vi "WPI_CANTalonSRX_Receive.vi"(11 "Device ID (0)":u8) -> (3 "Device ID":u8)   [LabVIEW 2016]
uses:
  <vilib>/Rock Robotics/WPI/ThirdParty/CanMotor/TalonSRX/WPI_CANTalonSRX_MessageIDs.ctl
  <vilib>/Rock Robotics/WPI/ThirdParty/CanMotor/TalonSRX/WPI_CANTalonSRX_GlobalOps.ctl
  <vilib>/Rock Robotics/WPI/ThirdParty/CanMotor/TalonSRX/WPI_CANTalonSRX_GlobalStatus.ctl
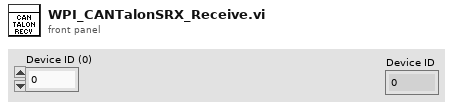
[diagram p1: front panel]
types:
  T1 = typedef "WPI_CANTalonSRX_MessageIDs.ctl" = u32
  T2 = typedef "WPI_CANTalonSRX_GlobalStatus.ctl" = cluster{"Applied Throttle":dbl, "Module Enabled":bool, "CAN Error":errorcluster, "Closed Loop Error":dbl, "Forward Limit Switch Closed":bool, "Reverse Limit Switch Closed":bool, "Sensor Position":dbl, "Sensor Velocity":dbl, "Current":dbl, "Sticky Fault - Over Temp":bool, "Sticky Fault - Under Voltage":bool, "Sticky Fault - Forward Limit":bool, "Sticky Fault - Reverse Limit":bool, "Sticky Fault - Forward Soft Limit":bool, "Sticky Fault - Reverse Soft Limit":bool, "Brake is Enabled":bool, "Encoder Position":dbl, "Encoder Velocity":dbl, "Encoder Index Count":dbl, "Encoder A Pin State":bool, "Encoder B Pin State":bool, "Encoder Index Pin State":bool, "Analog In":dbl, "Analog In Velocity":dbl, "Temperature (C)":dbl, "Battery Voltage":dbl, "Control 5 Is Supported":bool, "Current Profile Slot Select":dbl, "Pos Div 8":bool, "Vel Div 4":bool, "Pulse Width Position":i32, "Pulse Width Velocity":i32, "Pulse Width Rise To Rise (us)":i32, "Pulse Width Rise To Fall (us)":i32, "Mot Prof Active Is Under Run":bool, "Mot Prof Active Has Under Run":bool, "Mot Prof Active Is Last":bool, "Mot Prof Active Velocity Only":bool, "Mot Prof Active Is Valid":bool, "Mot Prof Buffer Is Full":bool, "Mot Prof Active Profile Slot Select":i32, "Mot Prof NextID":i32, "Mot Prof Count":i32, "Mot Prof Active Velocity":dbl, "Mot Prof Active Position":dbl, "Mot Prof Output Enable":i32, "UsageFrame":u32, "Motion Magic Active Trajectory":cluster{"Velocity":dbl, "Position":dbl}}
  T3 = typedef "WPI_CANTalonSRX_GlobalOps.ctl" = enum16{"Read For Send", "Write After Receive General", "Write After Receive Feedback", "Write After Receive Encoder", "Write After Receive Ain", "Write Error", "Get All", "Set Output", "Set Mode", "Set Master ID", "Set Brake Mode", "Set Reverse Feedback Sensor", "Set Reverse Closed Loop Output", "Set Override Limits", "Set Forward Limit Enabled", "Set Reverse Limit Enabled", "Set Feedback Select", "Set Profile Select", "Set Throttle Ramp Rate", "Disable", "Set Enc Codes Per Rev", "Set Num Pot Turns", "Set Control Frame Rate", "Enable Legacy Control", "Write After Receive Pulse Width", "Set Enable Frame Rate", "Write After Receive Motion Profile", "Set Motion Profile Flow Control", "Set Motion Profile Control Frame Rate", "Set Current Limit Enable", "Set Usage Frame", "Write After Receive Motion Magic"}
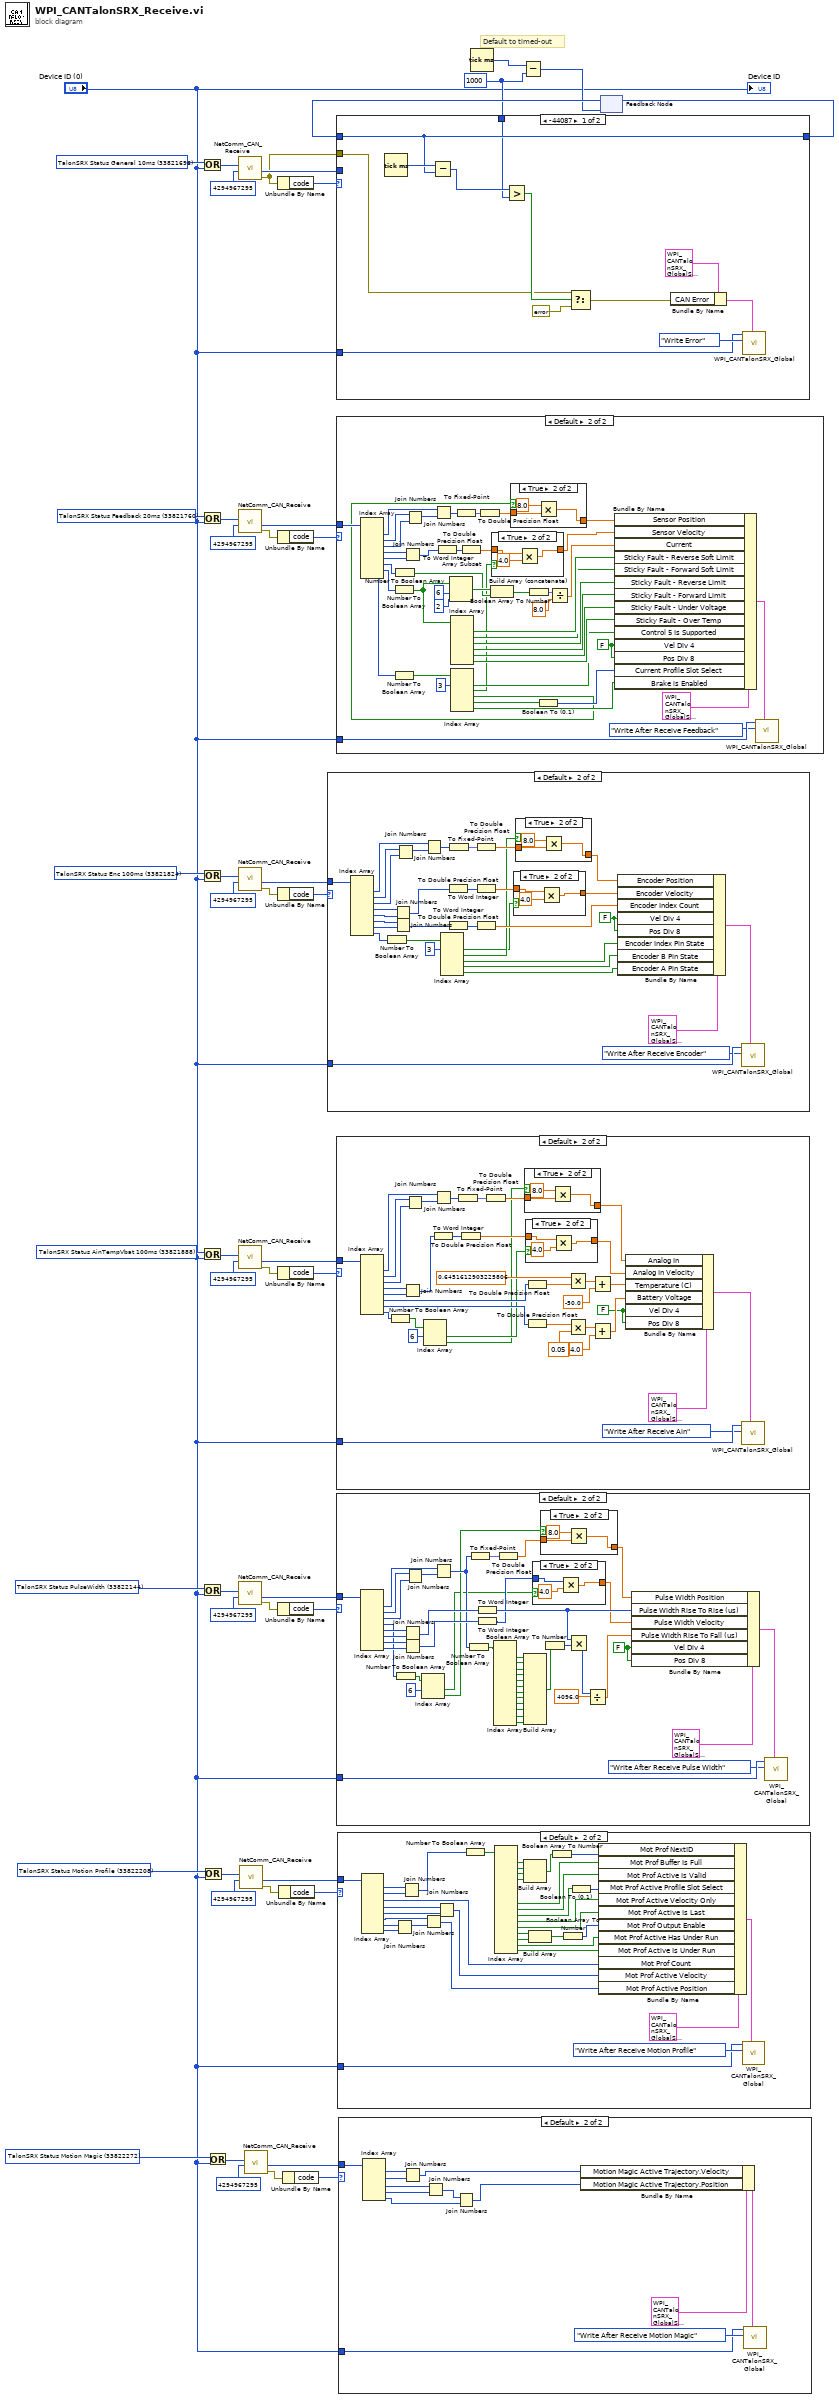
[diagram p0: block diagram]
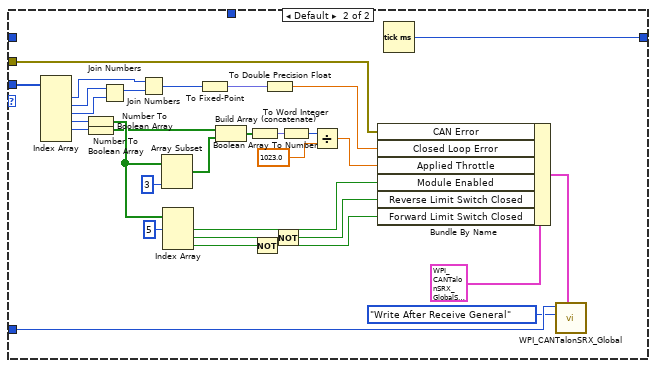
[diagram p16: hidden frame]
diagram:
  w2 = T1 33822272 items=["TalonSRX Control General 10ms"=33816576, "TalonSRX Control Rates Slow"=33816640, "TalonSRX Control ClearFlags Slow"=33816704, "TalonSRX Status General 10ms"=33821696, "TalonSRX Status Feedback 20ms"=33821760, "TalonSRX Status Enc 100ms"=33821824, "TalonSRX Status AinTempVbat 100ms"=33821888, "TalonSRX Status Startup Once"=33821952, "TalonSRX Status Debug"=33822080, "TalonSRX Config SetGainsSlot0 A"=33823808, "TalonSRX Config SetGainsSlot0 B"=33823872, "TalonSRX Config SetGainsSlot1 A"=33823936, "TalonSRX Config SetGainsSlot1 B"=33824000, "TalonSRX Config SetSoftLimits"=33824064, "TalonSRX Config WebControl"=33824128, "TalonSRX Param Request"=33822720, "TalonSRX Param Response"=33822784, "TalonSRX Param Set"=33822848, "TalonSRX Status PulseWidth"=33822144, "TalonSRX Status Motion Profile"=33822208, "TalonSRX Control General 5"=33816832, "TalonSRX Control Motion Profile Add"=33816896, "TalonSRX Status Motion Magic"=33822272] ("Talon SRX Control Frame")
  w8 = T1 33822208 items=["TalonSRX Control General 10ms"=33816576, "TalonSRX Control Rates Slow"=33816640, "TalonSRX Control ClearFlags Slow"=33816704, "TalonSRX Status General 10ms"=33821696, "TalonSRX Status Feedback 20ms"=33821760, "TalonSRX Status Enc 100ms"=33821824, "TalonSRX Status AinTempVbat 100ms"=33821888, "TalonSRX Status Startup Once"=33821952, "TalonSRX Status Debug"=33822080, "TalonSRX Config SetGainsSlot0 A"=33823808, "TalonSRX Config SetGainsSlot0 B"=33823872, "TalonSRX Config SetGainsSlot1 A"=33823936, "TalonSRX Config SetGainsSlot1 B"=33824000, "TalonSRX Config SetSoftLimits"=33824064, "TalonSRX Config WebControl"=33824128, "TalonSRX Param Request"=33822720, "TalonSRX Param Response"=33822784, "TalonSRX Param Set"=33822848, "TalonSRX Status PulseWidth"=33822144, "TalonSRX Status Motion Profile"=33822208, "TalonSRX Control General 5"=33816832, "TalonSRX Control Motion Profile Add"=33816896] ("Talon SRX Control Frame")
  w14 = T1 33822144 items=["TalonSRX Control General 10ms"=33816576, "TalonSRX Control Rates Slow"=33816640, "TalonSRX Control ClearFlags Slow"=33816704, "TalonSRX Status General 10ms"=33821696, "TalonSRX Status Feedback 20ms"=33821760, "TalonSRX Status Enc 100ms"=33821824, "TalonSRX Status AinTempVbat 100ms"=33821888, "TalonSRX Status Startup Once"=33821952, "TalonSRX Status Debug"=33822080, "TalonSRX Config SetGainsSlot0 A"=33823808, "TalonSRX Config SetGainsSlot0 B"=33823872, "TalonSRX Config SetGainsSlot1 A"=33823936, "TalonSRX Config SetGainsSlot1 B"=33824000, "TalonSRX Config SetSoftLimits"=33824064, "TalonSRX Config WebControl"=33824128, "TalonSRX Param Request"=33822720, "TalonSRX Param Response"=33822784, "TalonSRX Param Set"=33822848, "TalonSRX Status PulseWidth"=33822144, "TalonSRX Status Motion Profile"=33822208, "TalonSRX Control General 5"=33816832, "TalonSRX Control Motion Profile Add"=33816896] ("Talon SRX Control Frame")
  w21 = u32 1000 ("y")
  w27 = T1 33821888 items=["TalonSRX Control General 10ms"=33816576, "TalonSRX Control Rates Slow"=33816640, "TalonSRX Control ClearFlags Slow"=33816704, "TalonSRX Status General 10ms"=33821696, "TalonSRX Status Feedback 20ms"=33821760, "TalonSRX Status Enc 100ms"=33821824, "TalonSRX Status AinTempVbat 100ms"=33821888, "TalonSRX Status Startup Once"=33821952, "TalonSRX Status Debug"=33822080, "TalonSRX Config SetGainsSlot0 A"=33823808, "TalonSRX Config SetGainsSlot0 B"=33823872, "TalonSRX Config SetGainsSlot1 A"=33823936, "TalonSRX Config SetGainsSlot1 B"=33824000, "TalonSRX Config SetSoftLimits"=33824064, "TalonSRX Config WebControl"=33824128, "TalonSRX Param Request"=33822720, "TalonSRX Param Response"=33822784, "TalonSRX Param Set"=33822848]
  w34 = T1 33821824 items=["TalonSRX Control General 10ms"=33816576, "TalonSRX Control Rates Slow"=33816640, "TalonSRX Control ClearFlags Slow"=33816704, "TalonSRX Status General 10ms"=33821696, "TalonSRX Status Feedback 20ms"=33821760, "TalonSRX Status Enc 100ms"=33821824, "TalonSRX Status AinTempVbat 100ms"=33821888, "TalonSRX Status Startup Once"=33821952, "TalonSRX Status Debug"=33822080, "TalonSRX Config SetGainsSlot0 A"=33823808, "TalonSRX Config SetGainsSlot0 B"=33823872, "TalonSRX Config SetGainsSlot1 A"=33823936, "TalonSRX Config SetGainsSlot1 B"=33824000, "TalonSRX Config SetSoftLimits"=33824064, "TalonSRX Config WebControl"=33824128, "TalonSRX Param Request"=33822720, "TalonSRX Param Response"=33822784, "TalonSRX Param Set"=33822848]
  w39 = T1 33821760 items=["TalonSRX Control General 10ms"=33816576, "TalonSRX Control Rates Slow"=33816640, "TalonSRX Control ClearFlags Slow"=33816704, "TalonSRX Status General 10ms"=33821696, "TalonSRX Status Feedback 20ms"=33821760, "TalonSRX Status Enc 100ms"=33821824, "TalonSRX Status AinTempVbat 100ms"=33821888, "TalonSRX Status Startup Once"=33821952, "TalonSRX Status Debug"=33822080, "TalonSRX Config SetGainsSlot0 A"=33823808, "TalonSRX Config SetGainsSlot0 B"=33823872, "TalonSRX Config SetGainsSlot1 A"=33823936, "TalonSRX Config SetGainsSlot1 B"=33824000, "TalonSRX Config SetSoftLimits"=33824064, "TalonSRX Config WebControl"=33824128, "TalonSRX Param Request"=33822720, "TalonSRX Param Response"=33822784, "TalonSRX Param Set"=33822848]
  w46 = T1 33821696 items=["TalonSRX Control General 10ms"=33816576, "TalonSRX Control Rates Slow"=33816640, "TalonSRX Control ClearFlags Slow"=33816704, "TalonSRX Status General 10ms"=33821696, "TalonSRX Status Feedback 20ms"=33821760, "TalonSRX Status Enc 100ms"=33821824, "TalonSRX Status AinTempVbat 100ms"=33821888, "TalonSRX Status Startup Once"=33821952, "TalonSRX Status Debug"=33822080, "TalonSRX Config SetGainsSlot0 A"=33823808, "TalonSRX Config SetGainsSlot0 B"=33823872, "TalonSRX Config SetGainsSlot1 A"=33823936, "TalonSRX Config SetGainsSlot1 B"=33824000, "TalonSRX Config SetSoftLimits"=33824064, "TalonSRX Config WebControl"=33824128, "TalonSRX Param Request"=33822720, "TalonSRX Param Response"=33822784, "TalonSRX Param Set"=33822848]
  # "Default to timed-out"
  n1 = Or(x=w46, y="Device ID (0)") -> (x .or. y?=w47:T1)
  n2 = Or(x=w39, y="Device ID (0)") -> (x .or. y?=w38:T1)
  n3 = Or(x=w34, y="Device ID (0)") -> (x .or. y?=w35:T1)
  n4 = Or(x=w27, y="Device ID (0)") -> (x .or. y?=w26:T1)
  n5 = Or(x=w14, y="Device ID (0)") -> (x .or. y?=w18:T1)
  n6 = Or(x=w8, y="Device ID (0)") -> (x .or. y?=w12:T1)
  n7 = Or(x=w2, y="Device ID (0)") -> (x .or. y?=w5:T1)
  n8 = call <vilib>:"NetComm_CAN_Receive.vi"("Message ID Mask"=u32 4294967295, "Message ID"=w47) -> ("error out"=w44:errorcluster, "Data"=w48:u8[])  [unwired: 6 in, 2 out]
  n9 = call <vilib>:"NetComm_CAN_Receive.vi"("Message ID Mask"=u32 4294967295, "Message ID"=w38) -> ("error out"=w41:errorcluster, "Data"=w37:u8[])  [unwired: 6 in, 2 out]
  n10 = call <vilib>:"NetComm_CAN_Receive.vi"("Message ID Mask"=u32 4294967295, "Message ID"=w35) -> ("error out"=w32:errorcluster, "Data"=w36:u8[])  [unwired: 6 in, 2 out]
  n11 = call <vilib>:"NetComm_CAN_Receive.vi"("Message ID Mask"=u32 4294967295, "Message ID"=w26) -> ("error out"=w29:errorcluster, "Data"=w25:u8[])  [unwired: 6 in, 2 out]
  n12 = call <vilib>:"NetComm_CAN_Receive.vi"("Message ID Mask"=u32 4294967295, "Message ID"=w18) -> ("error out"=w16:errorcluster, "Data"=w19:u8[])  [unwired: 6 in, 2 out]
  n13 = call <vilib>:"NetComm_CAN_Receive.vi"("Message ID Mask"=u32 4294967295, "Message ID"=w12) -> ("error out"=w10:errorcluster, "Data"=w13:u8[])  [unwired: 6 in, 2 out]
  n14 = call <vilib>:"NetComm_CAN_Receive.vi"("Message ID Mask"=u32 4294967295, "Message ID"=w5) -> ("error out"=w7:errorcluster, "Data"=w4:u8[])  [unwired: 6 in, 2 out]
  n15 = Unbundle By Name(w44) -> ("code"=w43:i32)
  n16 = Unbundle By Name(w41) -> ("code"=w42:i32)
  n17 = Unbundle By Name(w32) -> ("code"=w31:i32)
  n18 = Unbundle By Name(w29) -> ("code"=w30:i32)
  n19 = Unbundle By Name(w16) -> ("code"=w15:i32)
  n20 = Unbundle By Name(w10) -> ("code"=w9:i32)
  n21 = Unbundle By Name(w7) -> ("code"=w3:i32)
  n22 = case shown="Default" w31 {
    tunnel: "Device ID (0)" -> [_ w81]
    tunnel: w36 -> [_ w80]
    frame -44087 {
    }
    frame Default {
      w49 = FALSE ("Vel Div 4")
      n23 = Index Array(array=w80) -> (element #1=w73:u8, element #2=w75:u8, element #3=w72:u8, element #4=w71:u8, element #5=w70:u8, element #6=w66:u8, element #7=w65:u8, element #8=w68:u8)  [unwired: 8 in]
      n24 = Number To Boolean Array(number=w68) -> (Boolean array=w78:bool[])
      n25 = Join Numbers(hi=w71, lo=w70) -> ((hi.lo)=w69:u16)
      n26 = Join Numbers(hi=w66, lo=w65) -> ((hi.lo)=w62:u16)
      n27 = Join Numbers(hi=w75, lo=w72) -> ((hi.lo)=w74:u16)
      n28 = Join Numbers(hi=w73, lo=w74) -> ((hi.lo)=w60:u32)
      n29 = Index Array(array=w78, index #1=3 ("index")) -> (element #1=w50:bool, element #2=w51:bool, element #3=w52:bool, element #4=w53:bool, element #5=w54:bool)  [unwired: 4 in]
      n30 = To Word Integer(number=w69) -> (16bit integer=w63:i16)
      n31 = To Word Integer(number=w62) -> (16bit integer=w61:i16)
      n32 = To Fixed-Point(number=w60) -> (fixed-point=w59:fxp<+/-,24,24>)  [unwired: 1 in]
      n33 = To Double Precision Float(number=w59) -> (double precision float=w57:dbl)
      n34 = To Double Precision Float(number=w63) -> (double precision float=w58:dbl)
      n35 = To Double Precision Float(number=w61) -> (double precision float=w67:dbl)
      n36 = case shown="True" w50 {
        tunnel: w58 -> [w82 w85]
        tunnel: [w82 w83] -> w56
        frame False {
        }
        frame True {
          n37 = Multiply(x=w85, y=4.0) -> (x*y=w83:dbl)
        }
      }
      n38 = case shown="True" w51 {
        tunnel: w57 -> [w86 w89]
        tunnel: [w86 w87] -> w55
        frame False {
        }
        frame True {
          n39 = Multiply(x=8.0, y=w89) -> (x*y=w87:dbl)
        }
      }
      n40 = Bundle By Name(cluster=T2 {"Applied Throttle"=0.0, "Module Enabled"=FALSE, "CAN Error"={"status"=FALSE, "code"=0, "source"=""}, "Closed Loop Error"=0.0, "Forward Limit Switch Closed"=FALSE, "Reverse Limit Switch Closed"=FALSE, "Sensor Position"=0.0, "Sensor Velocity"=0.0, "Current"=0.0, "Sticky Fault - Over Temp"=FALSE, "Sticky Fault - Under Voltage"=FALSE, "Sticky Fault - Forward Limit"=FALSE, "Sticky Fault - Reverse Limit"=FALSE, "Sticky Fault - Forward Soft Limit"=FALSE, "Sticky Fault - Reverse Soft Limit"=FALSE, "Brake is Enabled"=FALSE, "Encoder Position"=0.0, "Encoder Velocity"=0.0, "Encoder Index Count"=0.0, "Encoder A Pin State"=FALSE, "Encoder B Pin State"=FALSE, "Encoder Index Pin State"=FALSE, "Analog In"=0.0, "Analog In Velocity"=0.0, "Temperature (C)"=0.0, "Battery Voltage"=0.0, "Control 5 Is Supported"=FALSE, "Current Profile Slot Select"=0.0, "Pos Div 8"=FALSE, "Vel Div 4"=FALSE, "Pulse Width Position"=0, "Pulse Width Velocity"=0, "Pulse Width Rise To Rise (us)"=0, "Pulse Width Rise To Fall (us)"=0, "Mot Prof Active Is Under Run"=FALSE, "Mot Prof Active Has Under Run"=FALSE, "Mot Prof Active Is Last"=FALSE, "Mot Prof Active Velocity Only"=FALSE, "Mot Prof Active Is Valid"=FALSE, "Mot Prof Buffer Is Full"=FALSE, "Mot Prof Active Profile Slot Select"=0, "Mot Prof NextID"=0, "Mot Prof Count"=0, "Mot Prof Active Velocity"=0.0, "Mot Prof Active Position"=0.0, "Mot Prof Output Enable"=0, "UsageFrame"=0, "Motion Magic Active Trajectory"={"Velocity"=0.0, "Position"=0.0}} ("Write After Receive"), "Encoder Position"=w55, "Encoder Velocity"=w56, "Encoder Index Count"=w67, "Vel Div 4"=w49, "Pos Div 8"=w49, "Encoder Index Pin State"=w52, "Encoder B Pin State"=w53, "Encoder A Pin State"=w54) -> (w79:T2)
      n41 = call <vilib>:"WPI_CANTalonSRX_Global.vi"("Write After Receive"=w79, "Operation"=WPI_CANTalonSRX_GlobalOps."Write After Receive Encoder", "Device ID (0)"=w81) -> ()  [unwired: 6 in, 3 out]
    }
  }
  n42 = case shown="Default" w42 {
    tunnel: "Device ID (0)" -> [_ w135]
    tunnel: w37 -> [_ w134]
    frame -44087 {
    }
    frame Default {
      w90 = FALSE ("Vel Div 4")
      n43 = Index Array(array=w134) -> (element #1=w123:u8, element #2=w125:u8, element #3=w122:u8, element #4=w121:u8, element #5=w120:u8, element #6=w118:u8, element #7=w117:u8, element #8=w113:u8)  [unwired: 8 in]
      n44 = Number To Boolean Array(number=w117) -> (Boolean array=w132:bool[])
      n45 = Number To Boolean Array(number=w113) -> (Boolean array=w112:bool[])
      n46 = Number To Boolean Array(number=w118) -> (Boolean array=w103:bool[])
      n47 = Join Numbers(hi=w121, lo=w120) -> ((hi.lo)=w119:u16)
      n48 = Join Numbers(hi=w125, lo=w122) -> ((hi.lo)=w124:u16)
      n49 = Join Numbers(hi=w123, lo=w124) -> ((hi.lo)=w102:u32)
      n50 = To Word Integer(number=w119) -> (16bit integer=w105:i16)
      n51 = Array Subset(array=w132, index=6, length=2) -> (w104:bool[])
      n52 = Index Array(array=w132) -> (element #1=w110:bool, element #2=w109:bool, element #3=w108:bool, element #4=w107:bool, element #5=w106:bool, element #6=w111:bool)  [unwired: 6 in]
      n53 = Index Array(array=w112, index #1=3 ("index")) -> (element #1=w99:bool, element #2=w91:bool, element #3=w94:bool, element #4=w97:bool, element #5=w100:bool)  [unwired: 4 in]
      n54 = To Fixed-Point(number=w102) -> (fixed-point=w101:fxp<+/-,24,24>)  [unwired: 1 in]
      n55 = To Double Precision Float(number=w105) -> (double precision float=w93:dbl)
      n56 = To Double Precision Float(number=w101) -> (double precision float=w96:dbl)
      n57 = Build Array (concatenate)(w104, w103) -> (w130:bool[])
      n58 = case shown="True" w91 {
        tunnel: w93 -> [w136 w139]
        tunnel: [w136 w137] -> w92
        frame False {
        }
        frame True {
          n59 = Multiply(x=w139, y=4.0) -> (x*y=w137:dbl)
        }
      }
      n60 = case shown="True" w94 {
        tunnel: w96 -> [w140 w143]
        tunnel: [w140 w141] -> w95
        frame False {
        }
        frame True {
          n61 = Multiply(x=8.0, y=w143) -> (x*y=w141:dbl)
        }
      }
      n62 = Boolean Array To Number(Boolean array=w130) -> (number=w129:fxp<+/-,11,11>)
      n63 = Boolean To (0,1)(Boolean=w97) -> (0, 1=w98:i16)
      n64 = Divide(x=w129, y=8.0) -> (x/y=w115:dbl)
      n65 = Bundle By Name(cluster=T2 {"Applied Throttle"=0.0, "Module Enabled"=FALSE, "CAN Error"={"status"=FALSE, "code"=0, "source"=""}, "Closed Loop Error"=0.0, "Forward Limit Switch Closed"=FALSE, "Reverse Limit Switch Closed"=FALSE, "Sensor Position"=0.0, "Sensor Velocity"=0.0, "Current"=0.0, "Sticky Fault - Over Temp"=FALSE, "Sticky Fault - Under Voltage"=FALSE, "Sticky Fault - Forward Limit"=FALSE, "Sticky Fault - Reverse Limit"=FALSE, "Sticky Fault - Forward Soft Limit"=FALSE, "Sticky Fault - Reverse Soft Limit"=FALSE, "Brake is Enabled"=FALSE, "Encoder Position"=0.0, "Encoder Velocity"=0.0, "Encoder Index Count"=0.0, "Encoder A Pin State"=FALSE, "Encoder B Pin State"=FALSE, "Encoder Index Pin State"=FALSE, "Analog In"=0.0, "Analog In Velocity"=0.0, "Temperature (C)"=0.0, "Battery Voltage"=0.0, "Control 5 Is Supported"=FALSE, "Current Profile Slot Select"=0.0, "Pos Div 8"=FALSE, "Vel Div 4"=FALSE, "Pulse Width Position"=0, "Pulse Width Velocity"=0, "Pulse Width Rise To Rise (us)"=0, "Pulse Width Rise To Fall (us)"=0, "Mot Prof Active Is Under Run"=FALSE, "Mot Prof Active Has Under Run"=FALSE, "Mot Prof Active Is Last"=FALSE, "Mot Prof Active Velocity Only"=FALSE, "Mot Prof Active Is Valid"=FALSE, "Mot Prof Buffer Is Full"=FALSE, "Mot Prof Active Profile Slot Select"=0, "Mot Prof NextID"=0, "Mot Prof Count"=0, "Mot Prof Active Velocity"=0.0, "Mot Prof Active Position"=0.0, "Mot Prof Output Enable"=0, "UsageFrame"=0, "Motion Magic Active Trajectory"={"Velocity"=0.0, "Position"=0.0}} ("Write After Receive"), "Sensor Position"=w95, "Sensor Velocity"=w92, "Current"=w115, "Sticky Fault - Reverse Soft Limit"=w110, "Sticky Fault - Forward Soft Limit"=w109, "Sticky Fault - Reverse Limit"=w108, "Sticky Fault - Forward Limit"=w107, "Sticky Fault - Under Voltage"=w106, "Sticky Fault - Over Temp"=w111, "Control 5 Is Supported"=w99, "Vel Div 4"=w90, "Pos Div 8"=w90, "Current Profile Slot Select"=w98, "Brake is Enabled"=w100) -> (w133:T2)
      n66 = call <vilib>:"WPI_CANTalonSRX_Global.vi"("Write After Receive"=w133, "Operation"=WPI_CANTalonSRX_GlobalOps."Write After Receive Feedback", "Device ID (0)"=w135) -> ()  [unwired: 6 in, 3 out]
    }
  }
  n67 = case shown="Default" w30 {
    tunnel: "Device ID (0)" -> [_ w180]
    tunnel: w25 -> [_ w179]
    frame -44087 {
    }
    frame Default {
      w144 = FALSE ("Vel Div 4")
      n68 = Index Array(array=w179) -> (element #1=w173:u8, element #2=w175:u8, element #3=w172:u8, element #4=w171:u8, element #5=w170:u8, element #6=w166:u8, element #7=w167:u8, element #8=w153:u8)  [unwired: 8 in]
      n69 = Number To Boolean Array(number=w153) -> (Boolean array=w152:bool[])
      n70 = Join Numbers(hi=w171, lo=w170) -> ((hi.lo)=w169:u16)
      n71 = Join Numbers(hi=w175, lo=w172) -> ((hi.lo)=w174:u16)
      n72 = Index Array(array=w152, index #1=6 ("index")) -> (element #1=w146:bool, element #2=w145:bool)  [unwired: 1 in]
      n73 = To Word Integer(number=w169) -> (16bit integer=w156:i16)
      n74 = Join Numbers(hi=w173, lo=w174) -> ((hi.lo)=w155:u32)
      n75 = To Fixed-Point(number=w155) -> (fixed-point=w154:fxp<+/-,24,24>)  [unwired: 1 in]
      n76 = To Double Precision Float(number=w156) -> (double precision float=w148:dbl)
      n77 = To Double Precision Float(number=w154) -> (double precision float=w150:dbl)
      n78 = case shown="True" w145 {
        tunnel: w150 -> [w185 w188]
        tunnel: [w185 w186] -> w149
        frame False {
        }
        frame True {
          n79 = Multiply(x=8.0, y=w188) -> (x*y=w186:dbl)
        }
      }
      n80 = case shown="True" w146 {
        tunnel: w148 -> [w181 w184]
        tunnel: [w181 w182] -> w147
        frame False {
        }
        frame True {
          n81 = Multiply(x=w184, y=4.0) -> (x*y=w182:dbl)
        }
      }
      n82 = To Double Precision Float(number=w166) -> (double precision float=w157:dbl)
      n83 = To Double Precision Float(number=w167) -> (double precision float=w168:dbl)
      n84 = Multiply(x=0.6451612903225806, y=w157) -> (x*y=w161:dbl)
      n85 = Multiply(x=w168, y=0.05 ("x")) -> (x*y=w163:dbl)
      n86 = Add(x=w161, y=-50.0 ("x")) -> (x+y=w159:dbl)
      n87 = Add(x=w163, y=4.0 ("x")) -> (x+y=w165:dbl)
      n88 = Bundle By Name(cluster=T2 {"Applied Throttle"=0.0, "Module Enabled"=FALSE, "CAN Error"={"status"=FALSE, "code"=0, "source"=""}, "Closed Loop Error"=0.0, "Forward Limit Switch Closed"=FALSE, "Reverse Limit Switch Closed"=FALSE, "Sensor Position"=0.0, "Sensor Velocity"=0.0, "Current"=0.0, "Sticky Fault - Over Temp"=FALSE, "Sticky Fault - Under Voltage"=FALSE, "Sticky Fault - Forward Limit"=FALSE, "Sticky Fault - Reverse Limit"=FALSE, "Sticky Fault - Forward Soft Limit"=FALSE, "Sticky Fault - Reverse Soft Limit"=FALSE, "Brake is Enabled"=FALSE, "Encoder Position"=0.0, "Encoder Velocity"=0.0, "Encoder Index Count"=0.0, "Encoder A Pin State"=FALSE, "Encoder B Pin State"=FALSE, "Encoder Index Pin State"=FALSE, "Analog In"=0.0, "Analog In Velocity"=0.0, "Temperature (C)"=0.0, "Battery Voltage"=0.0, "Control 5 Is Supported"=FALSE, "Current Profile Slot Select"=0.0, "Pos Div 8"=FALSE, "Vel Div 4"=FALSE, "Pulse Width Position"=0, "Pulse Width Velocity"=0, "Pulse Width Rise To Rise (us)"=0, "Pulse Width Rise To Fall (us)"=0, "Mot Prof Active Is Under Run"=FALSE, "Mot Prof Active Has Under Run"=FALSE, "Mot Prof Active Is Last"=FALSE, "Mot Prof Active Velocity Only"=FALSE, "Mot Prof Active Is Valid"=FALSE, "Mot Prof Buffer Is Full"=FALSE, "Mot Prof Active Profile Slot Select"=0, "Mot Prof NextID"=0, "Mot Prof Count"=0, "Mot Prof Active Velocity"=0.0, "Mot Prof Active Position"=0.0, "Mot Prof Output Enable"=0, "UsageFrame"=0, "Motion Magic Active Trajectory"={"Velocity"=0.0, "Position"=0.0}} ("Write After Receive"), "Analog In"=w149, "Analog In Velocity"=w147, "Temperature (C)"=w159, "Battery Voltage"=w165, "Vel Div 4"=w144, "Pos Div 8"=w144) -> (w178:T2)
      n89 = call <vilib>:"WPI_CANTalonSRX_Global.vi"("Write After Receive"=w178, "Operation"=WPI_CANTalonSRX_GlobalOps."Write After Receive Ain", "Device ID (0)"=w180) -> ()  [unwired: 6 in, 3 out]
    }
  }
  n90 = case shown="Default" w15 {
    tunnel: "Device ID (0)" -> [_ w234]
    tunnel: w19 -> [_ w233]
    frame -44087 {
    }
    frame Default {
      w189 = FALSE ("Vel Div 4")
      n91 = Index Array(array=w233) -> (element #1=w227:u8, element #2=w229:u8, element #3=w226:u8, element #4=w198:u8, element #5=w222:u8, element #6=w221:u8, element #7=w220:u8, element #8=w219:u8)  [unwired: 8 in]
      n92 = Number To Boolean Array(number=w198) -> (Boolean array=w197:bool[])
      n93 = Join Numbers(hi=w222, lo=w221) -> ((hi.lo)=w225:u16)
      n94 = Join Numbers(hi=w220, lo=w219) -> ((hi.lo)=w224:u16)
      n95 = Join Numbers(hi=w229, lo=w226) -> ((hi.lo)=w228:u16)
      n96 = Index Array(array=w197, index #1=6 ("index")) -> (element #1=w190:bool, element #2=w191:bool)  [unwired: 1 in]
      n97 = Join Numbers(hi=w227, lo=w228) -> ((hi.lo)=w199:u32)
      n98 = Number To Boolean Array(number=w199) -> (Boolean array=w214:bool[])
      n99 = To Fixed-Point(number=w199) -> (fixed-point=w223:fxp<+/-,24,24>)  [unwired: 1 in]
      n100 = To Word Integer(number=w225) -> (16bit integer=w215:i16)
      n101 = To Word Integer(number=w224) -> (16bit integer=w193:i16)
      n102 = Index Array(array=w214) -> (element #1=w204:bool, element #2=w205:bool, element #3=w206:bool, element #4=w207:bool, element #5=w208:bool, element #6=w209:bool, element #7=w210:bool, element #8=w211:bool, element #9=w212:bool, element #10=w213:bool, element #11=w201:bool, element #12=w200:bool)  [unwired: 12 in]
      n103 = To Double Precision Float(number=w223) -> (double precision float=w194:dbl)
      n104 = Build Array(w204, w205, w206, w207, w208, w209, w210, w211, w212, w213, w201, w200) -> (w203:bool[])
      n105 = case shown="True" w190 {
        tunnel: w193 -> [w235 w238]
        tunnel: [w235 w236] -> w192
        frame False {
        }
        frame True {
          n106 = Multiply(x=w238, y=4.0) -> (x*y=w236:dbl)
        }
      }
      n107 = case shown="True" w191 {
        tunnel: w194 -> [w239 w242]
        tunnel: [w239 w240] -> w195
        frame False {
        }
        frame True {
          n108 = Multiply(x=8.0, y=w242) -> (x*y=w240:dbl)
        }
      }
      n109 = Boolean Array To Number(Boolean array=w203) -> (number=w202:u32)
      n110 = Multiply(x=w215, y=w202) -> (x*y=w217:u32)
      n111 = Divide(x=w217, y=4096.0) -> (x/y=w216:dbl)
      n112 = Bundle By Name(cluster=T2 {"Applied Throttle"=0.0, "Module Enabled"=FALSE, "CAN Error"={"status"=FALSE, "code"=0, "source"=""}, "Closed Loop Error"=0.0, "Forward Limit Switch Closed"=FALSE, "Reverse Limit Switch Closed"=FALSE, "Sensor Position"=0.0, "Sensor Velocity"=0.0, "Current"=0.0, "Sticky Fault - Over Temp"=FALSE, "Sticky Fault - Under Voltage"=FALSE, "Sticky Fault - Forward Limit"=FALSE, "Sticky Fault - Reverse Limit"=FALSE, "Sticky Fault - Forward Soft Limit"=FALSE, "Sticky Fault - Reverse Soft Limit"=FALSE, "Brake is Enabled"=FALSE, "Encoder Position"=0.0, "Encoder Velocity"=0.0, "Encoder Index Count"=0.0, "Encoder A Pin State"=FALSE, "Encoder B Pin State"=FALSE, "Encoder Index Pin State"=FALSE, "Analog In"=0.0, "Analog In Velocity"=0.0, "Temperature (C)"=0.0, "Battery Voltage"=0.0, "Control 5 Is Supported"=FALSE, "Current Profile Slot Select"=0.0, "Pos Div 8"=FALSE, "Vel Div 4"=FALSE, "Pulse Width Position"=0, "Pulse Width Velocity"=0, "Pulse Width Rise To Rise (us)"=0, "Pulse Width Rise To Fall (us)"=0, "Mot Prof Active Is Under Run"=FALSE, "Mot Prof Active Has Under Run"=FALSE, "Mot Prof Active Is Last"=FALSE, "Mot Prof Active Velocity Only"=FALSE, "Mot Prof Active Is Valid"=FALSE, "Mot Prof Buffer Is Full"=FALSE, "Mot Prof Active Profile Slot Select"=0, "Mot Prof NextID"=0, "Mot Prof Count"=0, "Mot Prof Active Velocity"=0.0, "Mot Prof Active Position"=0.0, "Mot Prof Output Enable"=0, "UsageFrame"=0, "Motion Magic Active Trajectory"={"Velocity"=0.0, "Position"=0.0}} ("Write After Receive"), "Pulse Width Position"=w195, "Pulse Width Rise To Rise (us)"=w215, "Pulse Width Velocity"=w192, "Pulse Width Rise To Fall (us)"=w216, "Vel Div 4"=w189, "Pos Div 8"=w189) -> (w232:T2)
      n113 = call <vilib>:"WPI_CANTalonSRX_Global.vi"("Write After Receive"=w232, "Operation"=WPI_CANTalonSRX_GlobalOps."Write After Receive Pulse Width", "Device ID (0)"=w234) -> ()  [unwired: 6 in, 3 out]
    }
  }
  n114 = case shown="Default" w9 {
    tunnel: w13 -> [_ w278]
    tunnel: "Device ID (0)" -> [_ w273]
    frame -44087 {
    }
    frame Default {
      n115 = Index Array(array=w278) -> (element #1=w266:u8, element #2=w265:u8, element #3=w243:u8, element #4=w268:u8, element #5=w269:u8, element #6=w272:u8, element #7=w271:u8, element #8=w270:u8)  [unwired: 8 in]
      n116 = Join Numbers(hi=w271, lo=w270) -> ((hi.lo)=w274:u16)
      n117 = Join Numbers(hi=w266, lo=w265) -> ((hi.lo)=w264:u16)
      n118 = Join Numbers(hi=w272, lo=w274) -> ((hi.lo)=w245:u32)
      n119 = Join Numbers(hi=w268, lo=w269) -> ((hi.lo)=w244:u16)
      n120 = Number To Boolean Array(number=w264) -> (Boolean array=w267:bool[])
      n121 = Index Array(array=w267) -> (element #1=w263:bool, element #2=w262:bool, element #3=w261:bool, element #4=w260:bool, element #8=w257:bool, element #9=w256:bool, element #10=w246:bool, element #11=w255:bool, element #12=w254:bool, element #13=w251:bool, element #14=w250:bool, element #15=w252:bool, element #16=w253:bool)  [unwired: 16 in, 3 out]
      n122 = Build Array(w263, w262, w261, w260) -> (w259:bool[])
      n123 = Build Array(w251, w250) -> (w248:bool[])
      n124 = Boolean Array To Number(Boolean array=w259) -> (number=w258:u32)
      n125 = Boolean Array To Number(Boolean array=w248) -> (number=w249:u32)
      n126 = Boolean To (0,1)(Boolean=w246) -> (0, 1=w247:i16)
      n127 = Bundle By Name(cluster=T2 {"Applied Throttle"=0.0, "Module Enabled"=FALSE, "CAN Error"={"status"=FALSE, "code"=0, "source"=""}, "Closed Loop Error"=0.0, "Forward Limit Switch Closed"=FALSE, "Reverse Limit Switch Closed"=FALSE, "Sensor Position"=0.0, "Sensor Velocity"=0.0, "Current"=0.0, "Sticky Fault - Over Temp"=FALSE, "Sticky Fault - Under Voltage"=FALSE, "Sticky Fault - Forward Limit"=FALSE, "Sticky Fault - Reverse Limit"=FALSE, "Sticky Fault - Forward Soft Limit"=FALSE, "Sticky Fault - Reverse Soft Limit"=FALSE, "Brake is Enabled"=FALSE, "Encoder Position"=0.0, "Encoder Velocity"=0.0, "Encoder Index Count"=0.0, "Encoder A Pin State"=FALSE, "Encoder B Pin State"=FALSE, "Encoder Index Pin State"=FALSE, "Analog In"=0.0, "Analog In Velocity"=0.0, "Temperature (C)"=0.0, "Battery Voltage"=0.0, "Control 5 Is Supported"=FALSE, "Current Profile Slot Select"=0.0, "Pos Div 8"=FALSE, "Vel Div 4"=FALSE, "Pulse Width Position"=0, "Pulse Width Velocity"=0, "Pulse Width Rise To Rise (us)"=0, "Pulse Width Rise To Fall (us)"=0, "Mot Prof Active Is Under Run"=FALSE, "Mot Prof Active Has Under Run"=FALSE, "Mot Prof Active Is Last"=FALSE, "Mot Prof Active Velocity Only"=FALSE, "Mot Prof Active Is Valid"=FALSE, "Mot Prof Buffer Is Full"=FALSE, "Mot Prof Active Profile Slot Select"=0, "Mot Prof NextID"=0, "Mot Prof Count"=0, "Mot Prof Active Velocity"=0.0, "Mot Prof Active Position"=0.0, "Mot Prof Output Enable"=0, "UsageFrame"=0, "Motion Magic Active Trajectory"={"Velocity"=0.0, "Position"=0.0}} ("Write After Receive"), "Mot Prof NextID"=w258, "Mot Prof Buffer Is Full"=w257, "Mot Prof Active Is Valid"=w256, "Mot Prof Active Profile Slot Select"=w247, "Mot Prof Active Velocity Only"=w255, "Mot Prof Active Is Last"=w254, "Mot Prof Output Enable"=w249, "Mot Prof Active Has Under Run"=w252, "Mot Prof Active Is Under Run"=w253, "Mot Prof Count"=w243, "Mot Prof Active Velocity"=w244, "Mot Prof Active Position"=w245) -> (w277:T2)
      n128 = call <vilib>:"WPI_CANTalonSRX_Global.vi"("Write After Receive"=w277, "Operation"=WPI_CANTalonSRX_GlobalOps."Write After Receive Motion Profile", "Device ID (0)"=w273) -> ()  [unwired: 6 in, 3 out]
    }
  }
  n129 = case shown="Default" w3 {
    tunnel: w4 -> [_ w291]
    tunnel: "Device ID (0)" -> [_ w287]
    frame -44087 {
    }
    frame Default {
      n130 = Index Array(array=w291) -> (element #1=w286:u8, element #2=w285:u8, element #3=w283:u8, element #4=w282:u8, element #5=w280:u8)  [unwired: 5 in]
      n131 = Join Numbers(hi=w286, lo=w285) -> ((hi.lo)=w284:u16)
      n132 = Join Numbers(hi=w283, lo=w282) -> ((hi.lo)=w281:u16)
      n133 = Join Numbers(hi=w281, lo=w280) -> ((hi.lo)=w279:u32)
      n134 = Bundle By Name(cluster=T2 {"Applied Throttle"=0.0, "Module Enabled"=FALSE, "CAN Error"={"status"=FALSE, "code"=0, "source"=""}, "Closed Loop Error"=0.0, "Forward Limit Switch Closed"=FALSE, "Reverse Limit Switch Closed"=FALSE, "Sensor Position"=0.0, "Sensor Velocity"=0.0, "Current"=0.0, "Sticky Fault - Over Temp"=FALSE, "Sticky Fault - Under Voltage"=FALSE, "Sticky Fault - Forward Limit"=FALSE, "Sticky Fault - Reverse Limit"=FALSE, "Sticky Fault - Forward Soft Limit"=FALSE, "Sticky Fault - Reverse Soft Limit"=FALSE, "Brake is Enabled"=FALSE, "Encoder Position"=0.0, "Encoder Velocity"=0.0, "Encoder Index Count"=0.0, "Encoder A Pin State"=FALSE, "Encoder B Pin State"=FALSE, "Encoder Index Pin State"=FALSE, "Analog In"=0.0, "Analog In Velocity"=0.0, "Temperature (C)"=0.0, "Battery Voltage"=0.0, "Control 5 Is Supported"=FALSE, "Current Profile Slot Select"=0.0, "Pos Div 8"=FALSE, "Vel Div 4"=FALSE, "Pulse Width Position"=0, "Pulse Width Velocity"=0, "Pulse Width Rise To Rise (us)"=0, "Pulse Width Rise To Fall (us)"=0, "Mot Prof Active Is Under Run"=FALSE, "Mot Prof Active Has Under Run"=FALSE, "Mot Prof Active Is Last"=FALSE, "Mot Prof Active Velocity Only"=FALSE, "Mot Prof Active Is Valid"=FALSE, "Mot Prof Buffer Is Full"=FALSE, "Mot Prof Active Profile Slot Select"=0, "Mot Prof NextID"=0, "Mot Prof Count"=0, "Mot Prof Active Velocity"=0.0, "Mot Prof Active Position"=0.0, "Mot Prof Output Enable"=0, "UsageFrame"=0, "Motion Magic Active Trajectory"={"Velocity"=0.0, "Position"=0.0}} ("Write After Receive"), "Motion Magic Active Trajectory.Velocity"=w284, "Motion Magic Active Trajectory.Position"=w279) -> (w290:T2)
      n135 = call <vilib>:"WPI_CANTalonSRX_Global.vi"("Write After Receive"=w290, "Operation"=WPI_CANTalonSRX_GlobalOps."Write After Receive Motion Magic", "Device ID (0)"=w287) -> ()  [unwired: 6 in, 3 out]
    }
  }
  n136 = Tick Count (ms)() -> (millisecond timer value=w22:u32)
  n137 = Subtract(x=w22, y=w21) -> (x-y=w20:u32)
  n138 = feedback #1(w20) -> (w23:u32)
  n139 = case shown="-44087" w43 {
    tunnel: "Device ID (0)" -> [w302 w334]
    tunnel: w48 -> [_ w333]
    tunnel: w44 -> [w295 w307]
    tunnel: [w298 w306] -> w24
    tunnel: w23 -> [w298 _]
    tunnel: w21 -> [w292 _]
    frame -44087 {
      n140 = Tick Count (ms)() -> (millisecond timer value=w299:u32)
      n141 = Subtract(x=w299, y=w298) -> (x-y=w297:u32)
      n142 = Greater?(x=w297, y=w292) -> (0:w296:bool)
      n143 = Select(t=w295, s=w296, f=errorcluster {"status"=FALSE, "code"=0, "source"=""}) -> (s? t:f=w294:errorcluster)
      n144 = Bundle By Name(cluster=T2 {"Applied Throttle"=0.0, "Module Enabled"=FALSE, "CAN Error"={"status"=FALSE, "code"=0, "source"=""}, "Closed Loop Error"=0.0, "Forward Limit Switch Closed"=FALSE, "Reverse Limit Switch Closed"=FALSE, "Sensor Position"=0.0, "Sensor Velocity"=0.0, "Current"=0.0, "Sticky Fault - Over Temp"=FALSE, "Sticky Fault - Under Voltage"=FALSE, "Sticky Fault - Forward Limit"=FALSE, "Sticky Fault - Reverse Limit"=FALSE, "Sticky Fault - Forward Soft Limit"=FALSE, "Sticky Fault - Reverse Soft Limit"=FALSE, "Brake is Enabled"=FALSE, "Encoder Position"=0.0, "Encoder Velocity"=0.0, "Encoder Index Count"=0.0, "Encoder A Pin State"=FALSE, "Encoder B Pin State"=FALSE, "Encoder Index Pin State"=FALSE, "Analog In"=0.0, "Analog In Velocity"=0.0, "Temperature (C)"=0.0, "Battery Voltage"=0.0, "Control 5 Is Supported"=FALSE, "Current Profile Slot Select"=0.0, "Pos Div 8"=FALSE, "Vel Div 4"=FALSE, "Pulse Width Position"=0, "Pulse Width Velocity"=0, "Pulse Width Rise To Rise (us)"=0, "Pulse Width Rise To Fall (us)"=0, "Mot Prof Active Is Under Run"=FALSE, "Mot Prof Active Has Under Run"=FALSE, "Mot Prof Active Is Last"=FALSE, "Mot Prof Active Velocity Only"=FALSE, "Mot Prof Active Is Valid"=FALSE, "Mot Prof Buffer Is Full"=FALSE, "Mot Prof Active Profile Slot Select"=0, "Mot Prof NextID"=0, "Mot Prof Count"=0, "Mot Prof Active Velocity"=0.0, "Mot Prof Active Position"=0.0, "Mot Prof Output Enable"=0, "UsageFrame"=0, "Motion Magic Active Trajectory"={"Velocity"=0.0, "Position"=0.0}} ("Write After Receive"), "CAN Error"=w294) -> (w300:T2)
      n145 = call <vilib>:"WPI_CANTalonSRX_Global.vi"("Write After Receive"=w300, "Operation"=WPI_CANTalonSRX_GlobalOps."Write Error", "Device ID (0)"=w302) -> ()  [unwired: 6 in, 3 out]
    }
    frame Default {
      n146 = Index Array(array=w333) -> (element #1=w314:u8, element #2=w317:u8, element #3=w313:u8, element #4=w329:u8, element #5=w326:u8)  [unwired: 6 in, 1 out]
      n147 = Number To Boolean Array(number=w329) -> (Boolean array=w328:bool[])
      n148 = Number To Boolean Array(number=w326) -> (Boolean array=w325:bool[])
      n149 = Join Numbers(hi=w317, lo=w313) -> ((hi.lo)=w316:u16)
      n150 = Join Numbers(hi=w314, lo=w316) -> ((hi.lo)=w315:u32)
      n151 = Array Subset(array=w328, length=3) -> (w324:bool[])  [unwired: 1 in]
      n152 = Index Array(array=w328, index #1=5 ("index")) -> (element #1=w330:bool, element #2=w309:bool, element #3=w308:bool)  [unwired: 2 in]
      n153 = To Fixed-Point(number=w315) -> (fixed-point=w311:fxp<+/-,24,24>)  [unwired: 1 in]
      n154 = Build Array (concatenate)(w325, w324) -> (w323:bool[])
      n155 = Boolean Array To Number(Boolean array=w323) -> (number=w322:fxp<+/-,11,11>)
      n156 = Not(x=w308) -> (.not. x?=w305:bool)
      n157 = To Double Precision Float(number=w311) -> (double precision float=w312:dbl)
      n158 = Not(x=w309) -> (.not. x?=w304:bool)
      n159 = To Word Integer(number=w322) -> (16bit integer=w310:i16)
      n160 = Divide(x=w310, y=1023.0) -> (x/y=w320:dbl)
      n161 = Bundle By Name(cluster=T2 {"Applied Throttle"=0.0, "Module Enabled"=FALSE, "CAN Error"={"status"=FALSE, "code"=0, "source"=""}, "Closed Loop Error"=0.0, "Forward Limit Switch Closed"=FALSE, "Reverse Limit Switch Closed"=FALSE, "Sensor Position"=0.0, "Sensor Velocity"=0.0, "Current"=0.0, "Sticky Fault - Over Temp"=FALSE, "Sticky Fault - Under Voltage"=FALSE, "Sticky Fault - Forward Limit"=FALSE, "Sticky Fault - Reverse Limit"=FALSE, "Sticky Fault - Forward Soft Limit"=FALSE, "Sticky Fault - Reverse Soft Limit"=FALSE, "Brake is Enabled"=FALSE, "Encoder Position"=0.0, "Encoder Velocity"=0.0, "Encoder Index Count"=0.0, "Encoder A Pin State"=FALSE, "Encoder B Pin State"=FALSE, "Encoder Index Pin State"=FALSE, "Analog In"=0.0, "Analog In Velocity"=0.0, "Temperature (C)"=0.0, "Battery Voltage"=0.0, "Control 5 Is Supported"=FALSE, "Current Profile Slot Select"=0.0, "Pos Div 8"=FALSE, "Vel Div 4"=FALSE, "Pulse Width Position"=0, "Pulse Width Velocity"=0, "Pulse Width Rise To Rise (us)"=0, "Pulse Width Rise To Fall (us)"=0, "Mot Prof Active Is Under Run"=FALSE, "Mot Prof Active Has Under Run"=FALSE, "Mot Prof Active Is Last"=FALSE, "Mot Prof Active Velocity Only"=FALSE, "Mot Prof Active Is Valid"=FALSE, "Mot Prof Buffer Is Full"=FALSE, "Mot Prof Active Profile Slot Select"=0, "Mot Prof NextID"=0, "Mot Prof Count"=0, "Mot Prof Active Velocity"=0.0, "Mot Prof Active Position"=0.0, "Mot Prof Output Enable"=0, "UsageFrame"=0, "Motion Magic Active Trajectory"={"Velocity"=0.0, "Position"=0.0}} ("Write After Receive"), "CAN Error"=w307, "Closed Loop Error"=w312, "Applied Throttle"=w320, "Module Enabled"=w330, "Reverse Limit Switch Closed"=w304, "Forward Limit Switch Closed"=w305) -> (w331:T2)
      n162 = Tick Count (ms)() -> (millisecond timer value=w306:u32)
      n163 = call <vilib>:"WPI_CANTalonSRX_Global.vi"("Write After Receive"=w331, "Operation"=WPI_CANTalonSRX_GlobalOps."Write After Receive General", "Device ID (0)"=w334) -> ()  [unwired: 6 in, 3 out]
    }
  }
  n164 = feedback-in #1(w24) -> ()
  "Device ID" <- "Device ID (0)"
